vi "5. Queue Based State Machine Traffic Light Simulator.vi"() -> ()   [LabVIEW 2018]
uses:
  Typedefs/Traffic Light States for Queue based example.ctl
panel:
  in  "stop":bool
  out "Yellow":bool
  out "Green":bool
  out "Red":bool
  out "Traffic Lights Picture":picture
  # "Traffic Light Graphic Vector by Vecteezy\n(https://www.vecteezy.com/free-vector/graphic)"
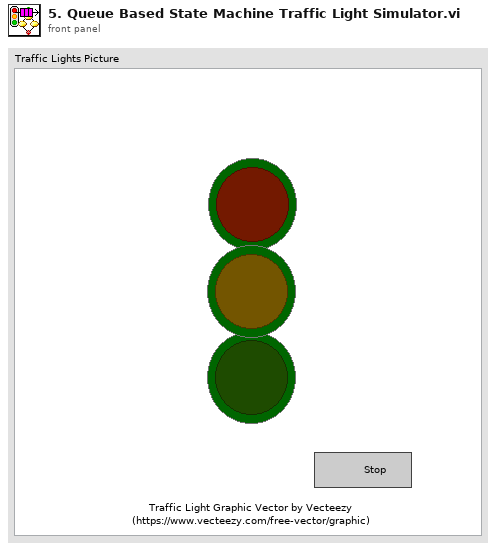
[diagram p1: front panel]
types:
  T1 = cluster{"Wait Before Red":u32, "Wait Before Yellow":u32, "Wait Before Green":u32}
  T2 = typedef "Traffic Light States for Queue based example.ctl" = enum16{"Initialize", "Red", "Yellow", "Green", "Wait", "Stop"}
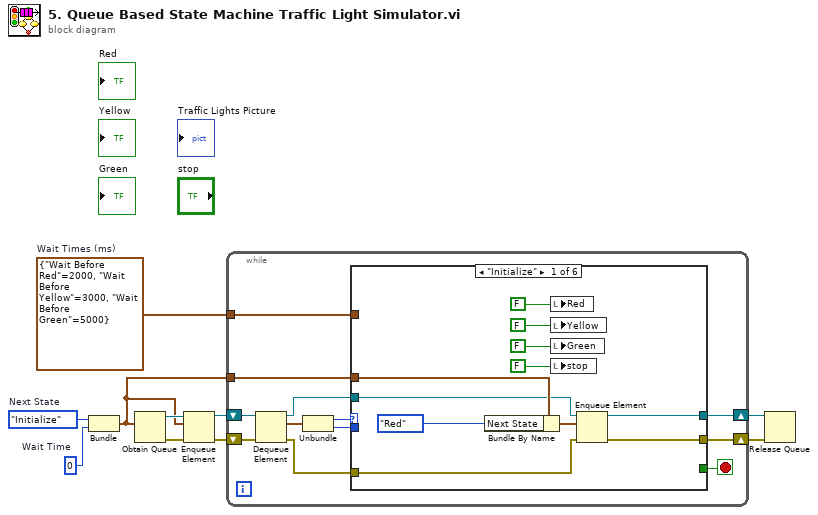
[diagram p0: block diagram]
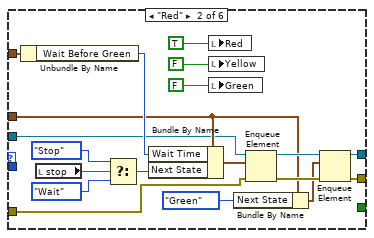
[diagram p2: hidden frame]
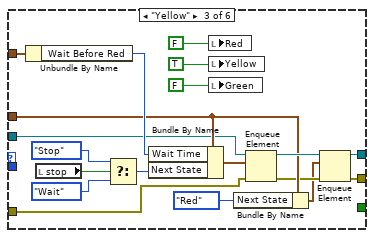
[diagram p3: hidden frame]
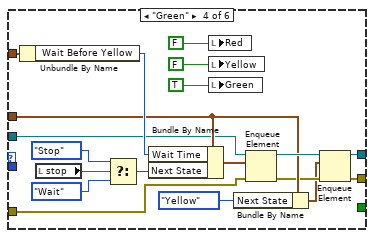
[diagram p4: hidden frame]
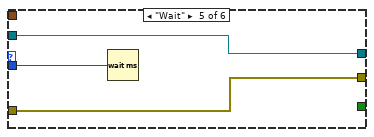
[diagram p5: hidden frame]
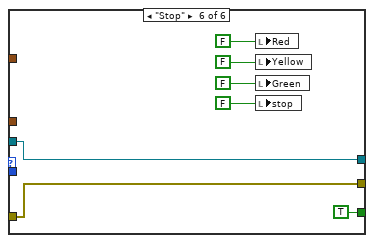
[diagram p6: hidden frame]
diagram:
  w8 = u32 0  # Wait Time
  w10 = T1 {"Wait Before Red"=2000, "Wait Before Yellow"=3000, "Wait Before Green"=5000}  # Wait Times (ms)
  w9 = Traffic_Light_States_for_Queue_based_example."Initialize"  # Next State
  n1 = Bundle("Next State"=w9, "Wait Time"=w8) -> (w4:cluster{"Next State":T2, "Wait Time":u32})  [unwired: 1 in]
  n2 = Obtain Queue(element data type=w4) -> (queue out=w7:refnum<queue>, error out=w5:errorcluster)  [unwired: 4 in, 1 out]
  n3 = Enqueue Element(queue=w7, element=w4, error in (no error)=w5) -> (queue out=w6:refnum<queue>, error out=w3:errorcluster)  [unwired: 1 in, 1 out]
  n4 = while {
    shift-right: [w16] -> w1
    shift-left: w6 -> [w20]
    tunnel: w10 -> [w22]
    tunnel: w4 -> [w17]
    shift-right: [w11] -> w2
    shift-left: w3 -> [w13]
    stop <- w21 stop-if-true
    n5 = Dequeue Element(queue=w20, error in (no error)=w13) -> (queue out=w15:refnum<queue>, element=w19:cluster{"Next State":T2, "Wait Time":u32}, error out=w12:errorcluster)  [unwired: 1 in, 1 out]
    n6 = Unbundle(w19) -> ("Next State"=w18:T2, "Wait Time"=w14:u32)
    n7 = case shown="\"Initialize\"" w18 {
      tunnel: [w26 w40 w60 w79 w93 w100] -> w16
      tunnel: w22 -> [_ w42 w62 w81 _ _]
      tunnel: [_ _ _ _ _ TRUE] -> w21
      tunnel: w17 -> [w29 w39 w59 w78 _ _]
      tunnel: w15 -> [w25 w36 w57 w76 w93 w100]
      tunnel: w14 -> [_ _ _ _ w92 _]
      tunnel: w12 -> [w24 w35 w56 w75 w91 w98]
      tunnel: [w23 w34 w53 w72 w91 w98] -> w11
      frame "Initialize" {
        n8 = Bundle By Name(cluster=w29, "Next State"=Traffic_Light_States_for_Queue_based_example."Red") -> (w27:cluster{"Next State":T2, "Wait Time":u32})
        n9 = local write "Red"(FALSE ("Red")) -> ()
        n10 = local write "Yellow"(FALSE ("Red")) -> ()
        n11 = local write "Green"(FALSE ("Red")) -> ()
        n12 = local write "stop"(FALSE ("stop")) -> ()
        n13 = Enqueue Element(queue=w25, element=w27, error in (no error)=w24) -> (queue out=w26:refnum<queue>, error out=w23:errorcluster)  [unwired: 1 in, 1 out]
      }
      frame "Red" {
        n14 = Unbundle By Name(w42) -> ("Wait Before Green"=w41:u32)
        n15 = local read "stop"() -> (w44:bool)
        n16 = Select(t=Traffic_Light_States_for_Queue_based_example."Stop" ("Next State"), s=w44, f=Traffic_Light_States_for_Queue_based_example."Wait" ("Next State")) -> (s? t:f=w45:T2)
        n17 = Bundle By Name(cluster=w39, "Wait Time"=w41, "Next State"=w45) -> (w48:cluster{"Next State":T2, "Wait Time":u32})
        n18 = local write "Red"(TRUE ("Red")) -> ()
        n19 = local write "Yellow"(FALSE ("Red")) -> ()
        n20 = local write "Green"(FALSE ("Red")) -> ()
        n21 = Bundle By Name(cluster=w39, "Next State"=Traffic_Light_States_for_Queue_based_example."Green") -> (w37:cluster{"Next State":T2, "Wait Time":u32})
        n22 = Enqueue Element(queue=w36, element=w48, error in (no error)=w35) -> (queue out=w47:refnum<queue>, error out=w52:errorcluster)  [unwired: 1 in, 1 out]
        n23 = Enqueue Element(queue=w47, element=w37, error in (no error)=w52) -> (queue out=w40:refnum<queue>, error out=w34:errorcluster)  [unwired: 1 in, 1 out]
      }
      frame "Yellow" {
        n24 = Unbundle By Name(w62) -> ("Wait Before Red"=w61:u32)
        n25 = local read "stop"() -> (w64:bool)
        n26 = Select(t=Traffic_Light_States_for_Queue_based_example."Stop" ("Next State"), s=w64, f=Traffic_Light_States_for_Queue_based_example."Wait" ("Next State")) -> (s? t:f=w65:T2)
        n27 = Bundle By Name(cluster=w59, "Wait Time"=w61, "Next State"=w65) -> (w68:cluster{"Next State":T2, "Wait Time":u32})
        n28 = local write "Red"(FALSE ("Red")) -> ()
        n29 = local write "Yellow"(TRUE ("Red")) -> ()
        n30 = local write "Green"(FALSE ("Red")) -> ()
        n31 = Bundle By Name(cluster=w59, "Next State"=Traffic_Light_States_for_Queue_based_example."Red") -> (w54:cluster{"Next State":T2, "Wait Time":u32})
        n32 = Enqueue Element(queue=w57, element=w68, error in (no error)=w56) -> (queue out=w67:refnum<queue>, error out=w55:errorcluster)  [unwired: 1 in, 1 out]
        n33 = Enqueue Element(queue=w67, element=w54, error in (no error)=w55) -> (queue out=w60:refnum<queue>, error out=w53:errorcluster)  [unwired: 1 in, 1 out]
      }
      frame "Green" {
        n34 = Unbundle By Name(w81) -> ("Wait Before Yellow"=w80:u32)
        n35 = local read "stop"() -> (w83:bool)
        n36 = Select(t=Traffic_Light_States_for_Queue_based_example."Stop" ("Next State"), s=w83, f=Traffic_Light_States_for_Queue_based_example."Wait" ("Next State")) -> (s? t:f=w84:T2)
        n37 = Bundle By Name(cluster=w78, "Wait Time"=w80, "Next State"=w84) -> (w87:cluster{"Next State":T2, "Wait Time":u32})
        n38 = local write "Red"(FALSE ("Red")) -> ()
        n39 = local write "Yellow"(FALSE ("Red")) -> ()
        n40 = local write "Green"(TRUE ("Red")) -> ()
        n41 = Bundle By Name(cluster=w78, "Next State"=Traffic_Light_States_for_Queue_based_example."Yellow") -> (w73:cluster{"Next State":T2, "Wait Time":u32})
        n42 = Enqueue Element(queue=w76, element=w87, error in (no error)=w75) -> (queue out=w86:refnum<queue>, error out=w74:errorcluster)  [unwired: 1 in, 1 out]
        n43 = Enqueue Element(queue=w86, element=w73, error in (no error)=w74) -> (queue out=w79:refnum<queue>, error out=w72:errorcluster)  [unwired: 1 in, 1 out]
      }
      frame "Wait" {
        n44 = Wait (ms)(milliseconds to wait=w92) -> ()  [unwired: 1 out]
      }
      frame "Stop" {
        n45 = local write "Red"(FALSE ("Red")) -> ()
        n46 = local write "Yellow"(FALSE ("Red")) -> ()
        n47 = local write "Green"(FALSE ("Red")) -> ()
        n48 = local write "stop"(FALSE ("stop")) -> ()
      }
    }
  }
  n49 = Release Queue(queue=w1, error in (no error)=w2) -> ()  [unwired: 1 in, 3 out]
